vi "Auto Get Seq Info from Server data.vi"(10 "SEQ Name":string, 11 "SEQ_Config":T1(array[cluster])) -> (2 "Acutal(T)/Reset(F)?":bool, 3 "Reset_SEQ":string[][](array[string]))   [LabVIEW 2020]
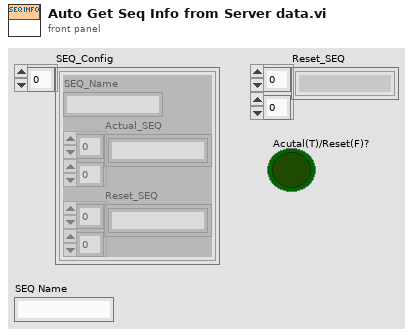
[diagram p1: front panel]
types:
  T1 = cluster{"SEQ_Name":string, "Actual_SEQ":string[][], "Reset_SEQ":string[][]}[]
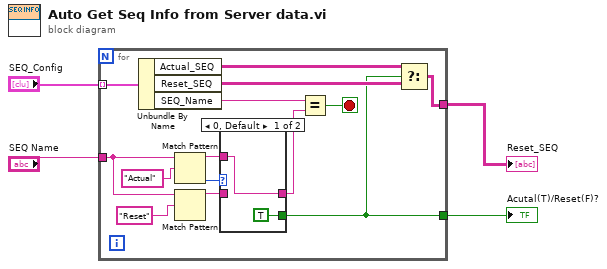
[diagram p0: block diagram]
diagram:
  n1 = for {
    tunnel: "SEQ_Config" -> [w18] mode=indexing
    tunnel: "SEQ Name" -> [w13]
    tunnel: [w8] -> w3
    tunnel: [w5] -> w2
    stop <- w16 stop-if-true
    n2 = Unbundle By Name(w18) -> ("Actual_SEQ"=w7:string[][], "Reset_SEQ"=w6:string[][], "SEQ_Name"=w17:string)
    n3 = Match Pattern(string=w13, regular expression="Actual") -> (before substring=w11:string, offset past match=w12:i32)  [unwired: 1 in, 2 out]
    n4 = Match Pattern(string=w13, regular expression="Reset") -> (before substring=w10:string)  [unwired: 1 in, 3 out]
    n5 = case shown="0, Default" w12 {
      tunnel: w11 -> [w20 _]
      tunnel: w10 -> [_ w21]
      tunnel: [w20 w21] -> w9
      tunnel: [TRUE _] -> w5
      frame 0, Default {
      }
      frame -1 {
      }
    }
    n6 = Equal?(x=w17, y=w9) -> (x = y?=w16:bool)
    n7 = Select(t=w7, s=w5, f=w6) -> (s? t:f=w8:string[][])
  }
  "Reset_SEQ" <- w3
  "Acutal(T)/Reset(F)?" <- w2
